vi "SetBgColorToBoolCtrl.vi"(10 "bg color":u32(colorbox)=65280, 11 "bool ref in":refnum<vi>) -> ()   [LabVIEW 2018, in "Library-Ctrl.lvlib"]
uses:
  Library-Ctrl.lvlib
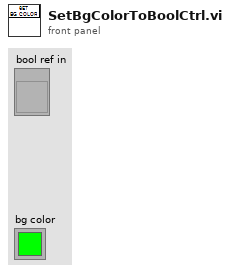
[diagram p1: front panel]
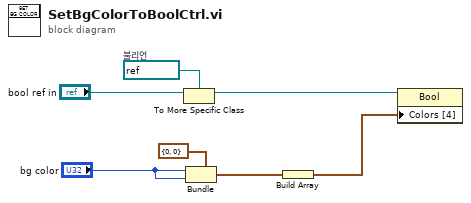
[diagram p0: block diagram]
diagram:
  w3 = refnum<vi> refnum  # 불리언
  n1 = To More Specific Class(target class=w3, reference="bool ref in") -> (specific class reference=w4:refnum<vi>)  [unwired: 1 in, 1 out]
  n2 = Bundle(cluster=cluster{u32, u32} {0, 0}, "bg color", "bg color") -> (w2:cluster{u32, u32})
  n3 = Build Array(w2) -> (w1:cluster{u32, u32}[])
  n4 = property class="Bool"(reference=w4, "Colors [4]"=w1) -> ()  [unwired: 1 in, 2 out]
